vi "AutoTurn.vi"(9 "Steady Val":dbl, 11 "Degrees to turn":dbl) -> ()   [LabVIEW 2012]
uses:
  State_Machine_Enum.ctl
  Robot Global Data.vi
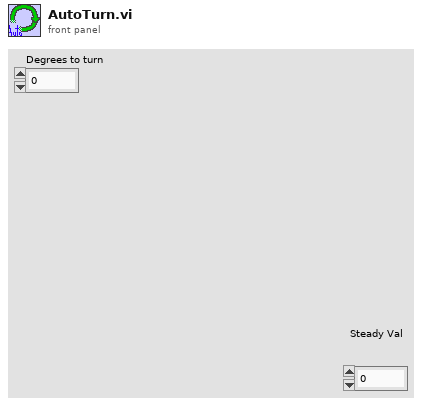
[diagram p1: front panel]
types:
  T1 = typedef "State_Machine_Enum.ctl" = enum16{"Idle", "Start", "Do", "Stop", "Init"}
  T2 = typedef "WPI_GyroDevRef.ctl" = cluster{"DevStatus":errorcluster, "Analog Module":T3, "Analog Channel":T4, "Offset":dbl, "Gain (VoltsPerDegree/Second)":dbl}
  T3 = typedef "FPGA_TypedefAnalogModule.ctl" = enum16{"Analog Module 1", "Analog Module 2"}
  T4 = typedef "FPGA_AIChannel.ctl" = enum8{"AI 1", "AI 2", "AI 3", "AI 4", "AI 5", "AI 6", "AI 7", "AI 8", "Invalid"}
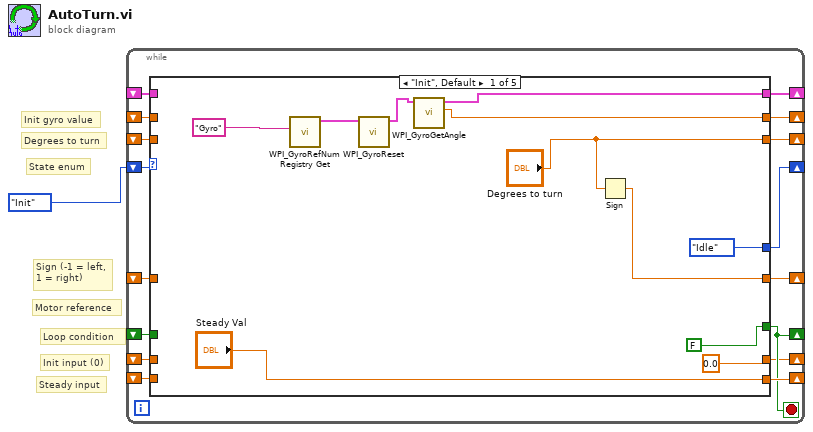
[diagram p0: block diagram]
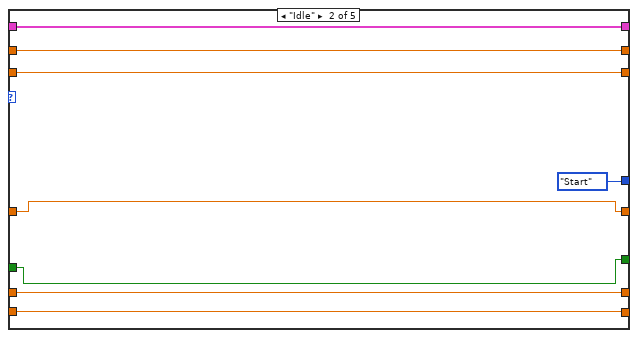
[diagram p2: hidden frame]
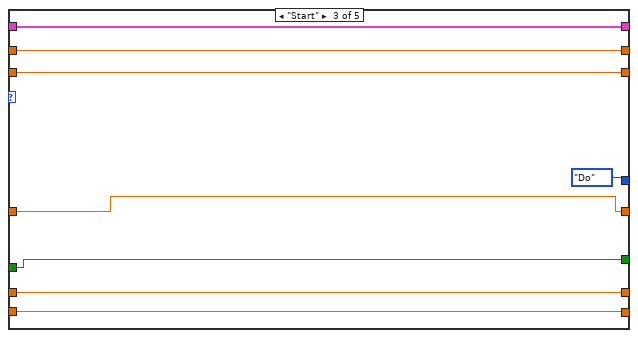
[diagram p3: hidden frame]
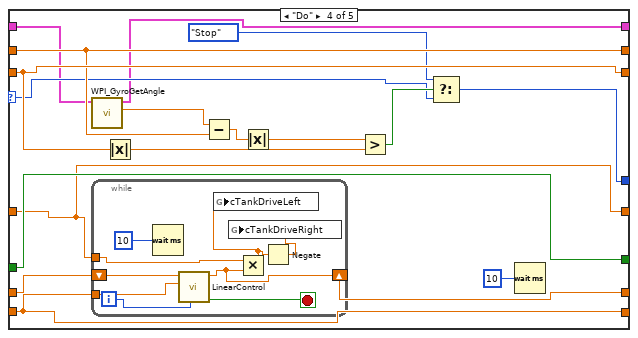
[diagram p4: hidden frame]
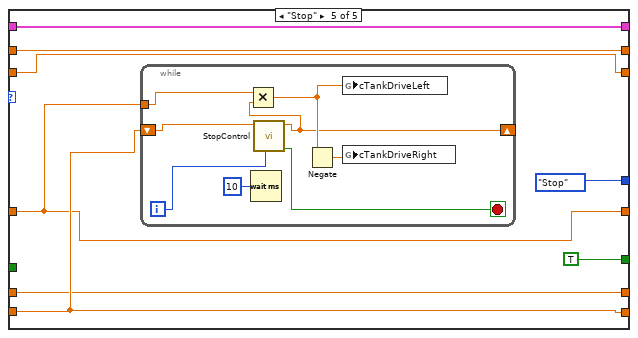
[diagram p5: hidden frame]
diagram:
  # "Sign (-1 = left,\n1 = right)"
  # "Degrees to turn"
  # "Init gyro value"
  # "State enum"
  # "Motor reference"
  # "Loop condition"
  # "Init input (0)"
  # "Steady input"
  n1 = while {
    shift-right: [w16] -> _
    shift-left: State_Machine_Enum."Init" ("State") -> [w17]
    shift-right: [w15] -> _
    shift-left: _ -> [w14]
    shift-right: [w13] -> _
    shift-left: _ -> [w12]
    shift-right: [w11] -> _
    shift-left: _ -> [w9]
    shift-right: [w10] -> _
    shift-left: _ -> [w8]
    shift-right: [w7] -> _
    shift-left: _ -> [w6]
    shift-right: [w5] -> _
    shift-left: _ -> [w4]
    shift-right: [w3] -> _
    shift-left: _ -> [w2]
    stop <- w13 stop-if-true
    n2 = case shown="\"Init\", Default" w17 {
      selector: w17 -> [_ _ _ w50 _]
      tunnel: [State_Machine_Enum."Idle" ("State") State_Machine_Enum."Start" ("State") State_Machine_Enum."Do" ("State") w62 State_Machine_Enum."Stop" ("State")] -> w16
      tunnel: ["Steady Val" w36 w44 w60 w79] -> w15
      tunnel: w14 -> [_ w36 w44 w60 w79]
      tunnel: [FALSE w35 w43 w59 TRUE] -> w13
      tunnel: w12 -> [_ w35 w43 w59 _]
      tunnel: [0.0 ("Right axis value") w34 w41 w56 w77] -> w11
      tunnel: [w18 w33 w42 w51 w76] -> w10
      tunnel: w9 -> [_ w34 w41 w57 w77]
      tunnel: w8 -> [_ w33 w42 w51 w76]
      tunnel: ["Degrees to turn" w32 w40 w52 w75] -> w7
      tunnel: w6 -> [_ w32 w40 w52 w75]
      tunnel: [w24 w31 w39 w49 w74] -> w5
      tunnel: w4 -> [_ w31 w39 w49 w74]
      tunnel: [w19 w29 w37 w45 w72] -> w3
      tunnel: w2 -> [_ w29 w37 w46 w72]
      frame "Init", Default {
        n3 = call <vilib>:"WPI_GyroRefNum Registry Get.vi"("refnum name"="Gyro") -> ("GyroDevRef"=w21:T2)  [unwired: 9 in, 1 out]
        n4 = call <vilib>:"WPI_GyroReset.vi"("GyroDevRef"=w21) -> ("GyroDevRef"=w20:T2)  [unwired: 9 in, 1 out]
        n5 = call <vilib>:"WPI_GyroGetAngle.vi"("GyroDevRef"=w20) -> ("Angle"=w18:dbl, "GyroDevRef"=w19:T2)  [unwired: 7 in, 2 out]
        n6 = Sign(1:"Degrees to turn") -> (0:w24:dbl)
      }
      frame "Idle" {
      }
      frame "Start" {
      }
      frame "Do" {
        n7 = call <vilib>:"WPI_GyroGetAngle.vi"("GyroDevRef"=w46) -> ("Angle"=w47:dbl, "GyroDevRef"=w45:T2)  [unwired: 7 in, 2 out]
        n8 = while {
          shift-right: [w64] -> w56
          shift-left: w57 -> [w71]
          tunnel: w60 -> [w67]
          tunnel: w49 -> [w70]
          i -> [w63]
          stop <- w65 stop-if-true
          n9 = Wait (ms)(milliseconds to wait=u32 10) -> ()  [unwired: 1 out]
          n10 = call "LinearControl.vi"("Loop Iteration"=w63, "Setpoint"=w67, "Motor Value"=w71) -> ("Currently Matching"=w65:bool, "New Motor Value"=w64:dbl)  [unwired: 7 in]
          n11 = Multiply(x=w70, y=w64) -> (x*y=w69:dbl)
          n12 = global write "Robot Global Data.vi" "cTankDriveLeft"(w69) -> ()
          n13 = Negate(x=w69) -> (-x=w68:dbl)
          n14 = global write "Robot Global Data.vi" "cTankDriveRight"(w68) -> ()
        }
        n15 = Absolute Value(x=w52) -> (abs(x)=w53:dbl)
        n16 = Subtract(x=w47, y=w51) -> (x-y=w55:dbl)
        n17 = Absolute Value(x=w55) -> (abs(x)=w54:dbl)
        n18 = Greater?(x=w54, y=w53) -> (0:w58:bool)
        n19 = Select(t=State_Machine_Enum."Stop" ("State"), s=w58, f=w50) -> (s? t:f=w62:T1)
        n20 = Wait (ms)(milliseconds to wait=u32 10) -> ()  [unwired: 1 out]
      }
      frame "Stop" {
        n21 = while {
          shift-right: [w82] -> _
          shift-left: w79 -> [w87]
          tunnel: w74 -> [w86]
          i -> [w80]
          stop <- w83 stop-if-true
          n22 = Wait (ms)(milliseconds to wait=u32 10) -> ()  [unwired: 1 out]
          n23 = call "StopControl.vi"("Loop Iteration"=w80, "Motor Value"=w87) -> ("Done Stopping"=w83:bool, "New Motor Value"=w82:dbl)  [unwired: 8 in]
          n24 = Multiply(x=w86, y=w82) -> (x*y=w84:dbl)
          n25 = Negate(x=w84) -> (-x=w85:dbl)
          n26 = global write "Robot Global Data.vi" "cTankDriveLeft"(w84) -> ()
          n27 = global write "Robot Global Data.vi" "cTankDriveRight"(w85) -> ()
        }
      }
    }
  }
